vi "CTRE_Phoenix_MotorController_Get_TalonFX.vi"   [LabVIEW 2020]
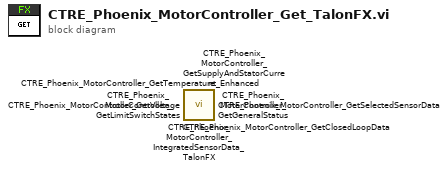
[diagram p0: block diagram]
diagram:
  n1 = call <vilib>:"CTRE_Phoenix_MotorController_IntegratedSensorData_TalonFX.vi"() -> ()  [unwired: 11 in, 5 out]
  n2 = call <vilib>:"CTRE_Phoenix_MotorController_GetSupplyAndStatorCurrent_Enhanced.vi"() -> ()  [unwired: 12 in, 4 out]
  n3 = call <vilib>:"CTRE_Phoenix_MotorController_GetLimitSwitchStates.vi"() -> ()  [unwired: 12 in, 4 out]
  n4 = call <vilib>:"CTRE_Phoenix_MotorController_GetGeneralStatus.vi"() -> ()  [unwired: 10 in, 6 out]
  n5 = call <vilib>:"CTRE_Phoenix_MotorController_GetTemperature.vi"() -> ()  [unwired: 13 in, 3 out]
  n6 = call <vilib>:"CTRE_Phoenix_MotorController_GetClosedLoopData.vi"() -> ()  [unwired: 10 in, 6 out]
  n7 = call <vilib>:"CTRE_Phoenix_MotorController_GetSelectedSensorData.vi"() -> ()  [unwired: 12 in, 4 out]
  n8 = call <vilib>:"CTRE_Phoenix_MotorController_GetVoltage.vi"() -> ()  [unwired: 11 in, 5 out]
